vi "Stanford Research 844 Display Data Measurement.vi"(0 "VISA Resource Name":refnum<visa-resource-name>, 1 "Channel 1 Display (0: X)":u16(ring) items=["X", "R [Volts rms]", "R [dBm]", "X noise", "AUX IN 1"], 2 "Channel 2 Display (0: Y)":u16(ring) items=["Y", "Phi", "Y noise [Volts]", "Y noise [dBm]", "AUX IN 2"], 7 "Parameters (0: X, 1: Y)":i32[](array[ring])=[0, 1, 2, 4, 8, 9] items=["X", "Y", "R [V]", "R [dBm]", "Phi", "AUX IN 1", "AUX IN 2", "Reference Frequency", "CH1 Display", "CH2 Display"]) -> (6 "Channel 1 Display Value":dbl format="%.5p", 8 "Channel 2 Display Value":dbl format="%.5p", 10 "Corresponding Values":dbl[](array[numeric]) format="%.5e")   [LabVIEW 2010]
doc: "This VI shows basic of operations of instrument - how to read value(s) from instrument."
uses:
  <instrlib>/Stanford Research 844/Stanford Research 844.lvlib
panel:
  # "© 2005 National Instruments.  ALL RIGHTS RESERVED."
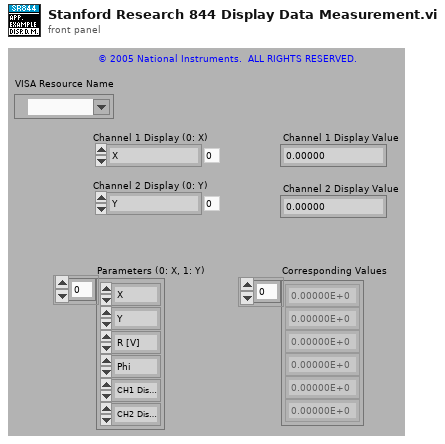
[diagram p1: front panel]
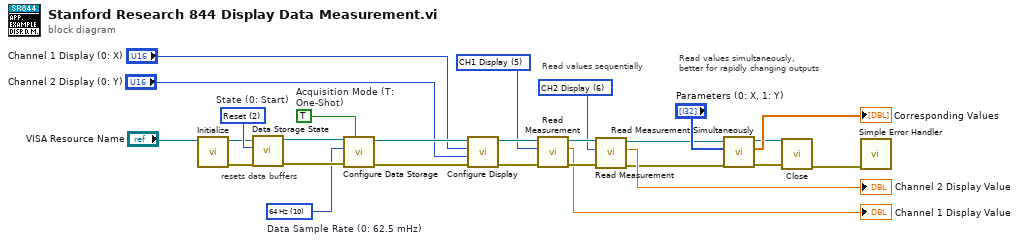
[diagram p0: block diagram]
diagram:
  w7 = TRUE  # Acquisition Mode (T: One-Shot)
  w8 = u16 6 items=["X", "Y", "R [V]", "R [dBm]", "Phi", "CH1 Display", "CH2 Display", "AUX 1", "AUX 2"] ("Value Selection (0: X)")
  w10 = u16 5 items=["X", "Y", "R [V]", "R [dBm]", "Phi", "CH1 Display", "CH2 Display", "AUX 1", "AUX 2"] ("Value Selection (0: X)")
  w24 = u16 10 items=["62.5 mHz", "125 mHz", "250 mHz", "500 mHz", "1 Hz", "2 Hz", "4 Hz", "8 Hz", "16 Hz", "32 Hz", "64 Hz", "128 Hz", "256 Hz", "512 Hz", "Trigger"]  # Data Sample Rate (0: 62.5 mHz)
  w27 = u16 2 items=["Start", "Pause", "Reset"]  # State (0: Start)
  # "resets data buffers"
  # "Read values sequentially"
  # "Read values simultaneously, \nbetter for rapidly changing outputs"
  n1 = call <instrlib>:"Initialize.vi"("VISA Resource Name"="VISA Resource Name") -> ("error out"=w5:errorcluster, "VISA Resource Name Out"=w6:refnum<visa-resource-name>)  [unwired: 9 in]
  n2 = call <instrlib>:"Data Storage State.vi"("Error In (no error)"=w5, "State (0: Start)"=w27, "VISA Resource Name"=w6) -> ("Error Out"=w25:errorcluster, "VISA Resource Name Out"=w26:refnum<visa-resource-name>)  [unwired: 7 in]
  n3 = call <instrlib>:"Configure Data Storage.vi"("Acquisition Mode (T: One-Shot)"=w7, "Error In (no error)"=w25, "Data Sample Rate (0: 62.5 mHz)"=w24, "VISA Resource Name"=w26) -> ("Error Out"=w22:errorcluster, "VISA Resource Name Out"=w23:refnum<visa-resource-name>)  [unwired: 6 in]
  n4 = call <instrlib>:"Configure Display.vi"("Error In (no error)"=w22, "Channel 2 Display (0: Y)"="Channel 2 Display (0: Y)", "Channel 1 Display (0: X)"="Channel 1 Display (0: X)", "VISA Resource Name"=w23) -> ("Error Out"=w18:errorcluster, "VISA Resource Name Out"=w19:refnum<visa-resource-name>)  [unwired: 6 in]
  n5 = call <instrlib>:"Read Measurement.vi"("Error In (no error)"=w18, "Value Selection (0: X)"=w10, "VISA Resource Name"=w19) -> ("Error Out"=w16:errorcluster, "Value"=→"Channel 1 Display Value":dbl, "VISA Resource Name Out"=w17:refnum<visa-resource-name>)  [unwired: 6 in]
  n6 = call <instrlib>:"Read Measurement.vi"("Error In (no error)"=w16, "Value Selection (0: X)"=w8, "VISA Resource Name"=w17) -> ("Error Out"=w12:errorcluster, "Value"=→"Channel 2 Display Value":dbl, "VISA Resource Name Out"=w13:refnum<visa-resource-name>)  [unwired: 6 in]
  n7 = call <instrlib>:"Read Measurement Simultaneously.vi"("Error In (no error)"=w12, "Parameters (0: X, 1: Y)"="Parameters (0: X, 1: Y)", "VISA Resource Name"=w13) -> ("Error Out"=w3:errorcluster, "Values"=→"Corresponding Values":dbl[], "VISA Resource Name Out"=w2:refnum<visa-resource-name>)  [unwired: 6 in]
  n8 = call <instrlib>:"Close.vi"("error in (no error)"=w3, "VISA Resource Name"=w2) -> ("error out"=w1:errorcluster)  [unwired: 9 in]
  n9 = call <vilib>:"Simple Error Handler.vi"("error in (no error)"=w1) -> ()  [unwired: 4 in, 5 out]
